vi "VMS.vi"(0 "PhoneNumbers":string, 5 "内容":string, 11 "error in (no error)":errorcluster caption="错误输入（无错误）") -> (4 "headers":string caption="头部", 6 "body":string caption="体部", 15 "error out":errorcluster caption="错误输出")   [LabVIEW 2016]
uses:
  <vilib>/LVH/i3 JSON/JSON Generation/Create Value Files/Create Value - String.vi
  <vilib>/LVH/i3 OAuth/i3-oauth.lvlib
  <vilib>/httpClient/LabVIEWHTTPClient.lvlib
  <vilib>/LVH/i3 JSON/i3-json.lvlib
panel:
  out "GET String":string
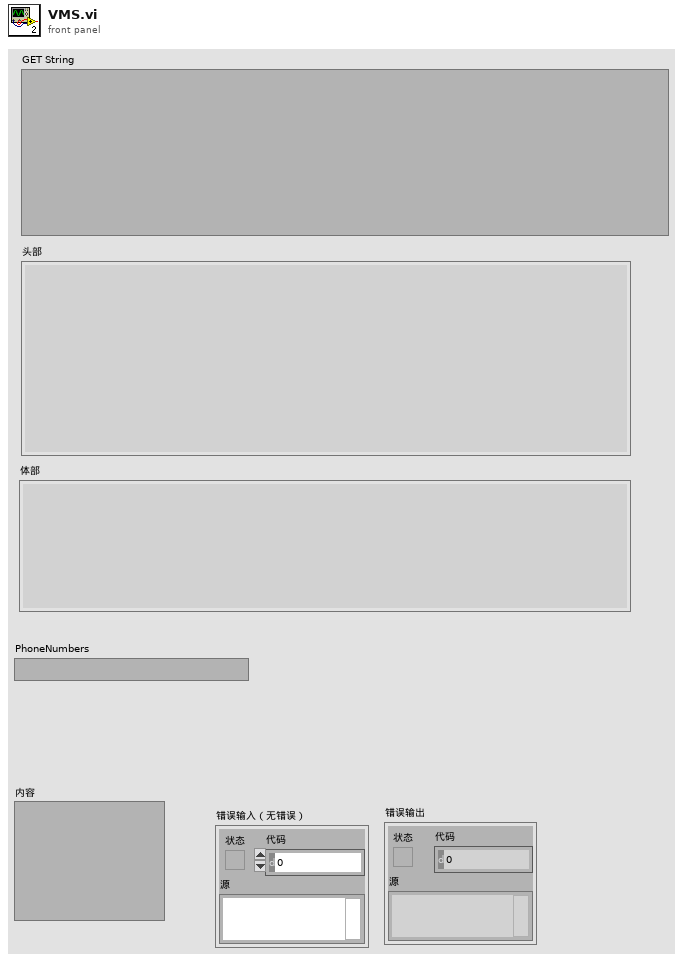
[diagram p1: front panel]
types:
  T1 = cluster{"Action":string, "CalledNumber":string, "CalledShowNumber":string, "TtsCode":string, "TtsParam":string, "PlayTimes":string, "Volume":string, "Speed":string, "OutId":string, "Version":string}
  T2 = cluster{"AccessKeyId":string, "Timestamp":string, "Format":string, "SignatureMethod":string, "SignatureVersion":string, "SignatureNonce":string, "Signature":string}
  T3 = typedef "i3-oauth.lvlib/Name-Value Pair.ctl" = cluster{"Name":string, "Value":string}
  T4 = typedef "LabVIEWHTTPClient.lvlib/ClientHandle.ctl" = refnum<k1>
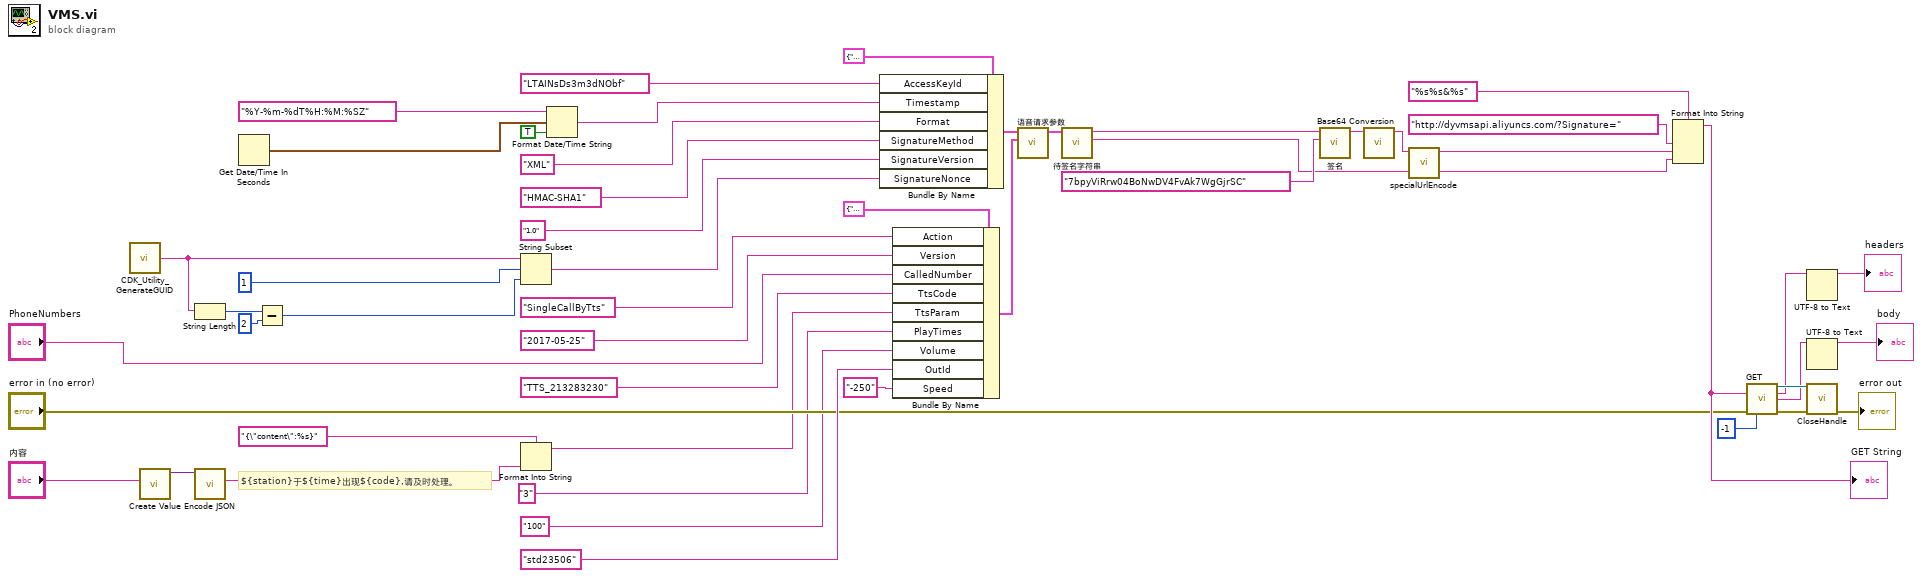
[diagram p0: block diagram]
diagram:
  # "${station}于${time}出现${code},请及时处理。"
  n1 = call <resource>:"CDK_Utility_GenerateGUID.vi"() -> ("GUID"=w33:string)  [unwired: 9 in]
  n2 = call-poly <vilib>:"Create Value.vi"("String"="内容") -> ("JSON Tree"=w18:variant)  [unwired: 9 in, 1 out]
  n3 = String Length(string=w33) -> (length=w32:i32)
  n4 = call <vilib>:"Encode JSON.vi"("JSON Tree"=w18) -> ("String"=w14:string)  [unwired: 5 in, 1 out]
  n5 = Get Date/Time In Seconds() -> (seconds since 1Jan1904=w28:timestamp)
  n6 = Subtract(x=w32, y=2) -> (x-y=w30:i32)
  n7 = String Subset(string=w33, offset (0)=1 ("偏移量(0)"), length (rest)=w30) -> (substring=w29:string)
  n8 = Format Into String(format string="{\"content\":%s}" ("TemplateParam"), w14) -> (resulting string=w5:string)  [unwired: 2 in, 1 out]
  n9 = Format Date/Time String(time format string (%c)="%Y-%m-%dT%H:%M:%SZ" ("时间格式字符串(%c)"), seconds (now)=w28, UTC format=TRUE ("UTC格式")) -> (date/time string=w25:string)
  n10 = Bundle By Name(cluster=T2 {"AccessKeyId"="", "Timestamp"="", "Format"="", "SignatureMethod"="", "SignatureVersion"="", "SignatureNonce"="", "Signature"=""} ("系统参数"), "AccessKeyId"="LTAINsDs3m3dNObf", "Timestamp"=w25, "Format"="XML", "SignatureMethod"="HMAC-SHA1", "SignatureVersion"="1.0", "SignatureNonce"=w29) -> (w42:T2)
  n11 = Bundle By Name(cluster=T1 {"Action"="", "CalledNumber"="", "CalledShowNumber"="", "TtsCode"="", "TtsParam"="", "PlayTimes"="", "Volume"="", "Speed"="", "OutId"="", "Version"=""} ("业务参数"), "Action"="SingleCallByTts", "Version"="2017-05-25", "CalledNumber"="PhoneNumbers", "TtsCode"="TTS_213283230", "TtsParam"=w5, "PlayTimes"="3", "Volume"="100", "OutId"="std23506", "Speed"="-250") -> (w1:T1)
  n12 = call "语音请求参数.vi"("业务参数"=w1, "系统参数"=w42) -> ("已排序的数组"=w50:T3[])  [unwired: 9 in]
  n13 = call "待签名字符串.vi"("已排序的数组"=w50) -> ("sortQueryString"=w22:string, "StringToSign"=w38:string)  [unwired: 9 in]
  n14 = call "签名.vi"("consumer secret"="7bpyViRrw04BoNwDV4FvAk7WgGjrSC", "Signature Base string"=w38) -> ("Encoded Signature"=w48:string)  [unwired: 9 in]
  n15 = call <vilib>:"Base64 Conversion.vi"("String"=w48) -> ("Base64 String"=w35:string)  [unwired: 10 in]
  n16 = call "specialUrlEncode.vi"("str"=w35) -> ("UrlEncode"=w23:string)  [unwired: 10 in]
  n17 = Format Into String(format string="%s%s&%s" ("格式字符串"), "http://dyvmsapi.aliyuncs.com/?Signature=" ("输入 1"), w23, w22) -> (resulting string=w24:string)  [unwired: 2 in, 1 out]
  "GET String" <- w24
  n18 = call <vilib>:"GET.vi"("url"=w24, "error in (no error)"="error in (no error)", "timeout (10000)"=-1) -> ("client handle out"=w21:T4, "headers"=w11:string, "body"=w13:string, "error out"=w20:errorcluster)  [unwired: 9 in]
  n19 = UTF-8 to Text(11:w11) -> (3:→"headers":string)  [unwired: 2 in, 1 out]
  n20 = UTF-8 to Text(11:w13) -> (3:→"body":string)  [unwired: 2 in, 1 out]
  n21 = call <vilib>:"CloseHandle.vi"("client handle"=w21, "error in (no error)"=w20) -> ("error out"=→"error out":errorcluster)  [unwired: 13 in]
